vi "RasterScanXY.vi"(4 "Scanning parameters":T1) -> (1 "X,Y AO Waveforms":waveform(dbl)[](array[waveform]))   [LabVIEW 2015]
doc: "DESCRIPTION:\nThis example generates a sinewave analog output waveform on the board specified. It is an example of the simplest form of continuous waveform generation. \nA sine wave is computed using the sine trig function in a for loop. The analog output channel and buffer is initialized (AO Config), the waveform written to the the waveform buffer (AO Write) and waveform generation is initiated at the specified update rate (AO Start).\n\n\nINSTRUCTIONS:\n1. Specify device, channels, and update rate.\n2. If you want the waveform to be regenerated indefinitely, set cycles to generate to 0. Otherwise, specify the cycles to generate as a positive number. \n3. Run the VI. You will see the number of cycles generated in the cycles done indicator.\n4. If no error occurred, the example waits in a while loop for the stop button to be pressed or the requested number of buffer iterations to be completed. When either condition occurs, AO Clear stops the wavefrom generation.\n\n\nKEY PARAMETERS:\n* AO Config: device, channel\n* AO Write: (sinewave data)\n* AO Start: update rate, cycles to generate\n\n \nI/O CONNECTIONS OVERVIEW:\nConnect the I/O connector pin of the specified analog output channel to an external device (e.g. oscilloscope).\n\n\nModification Ideas:\n- For multiple channel waveform generation:\nSimply compute waveforms for other channels and collect them in a 2D array - one row for each channel. Then transpose the 2D array before connecting to AO Write. Enter the multiple channels in the \"channel\" control.\n\n- To change the waveform during generation:\nAO Write can also be used in the loop to update the waveform buffer. See the Function Generator example."
panel:
  # "this correspondes to channel \n\"0\" in stage"
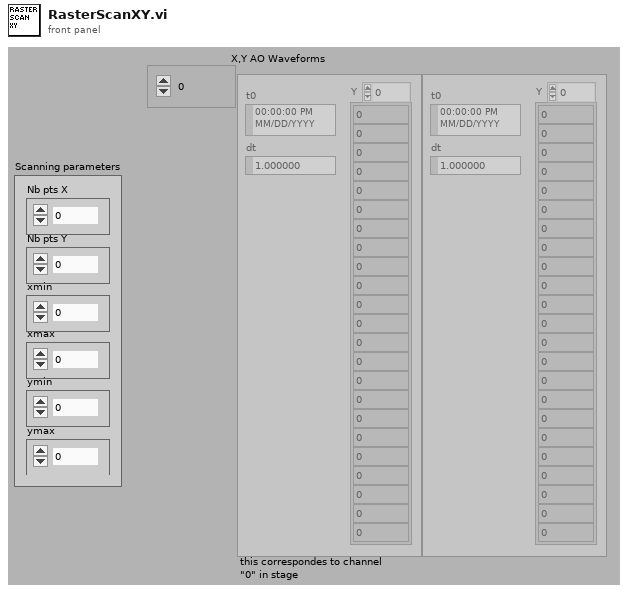
[diagram p1: front panel]
types:
  T1 = cluster{"Nb pts X":u32, "Nb pts Y":u32, "xmin":dbl, "xmax":dbl, "ymin":dbl, "ymax":dbl}
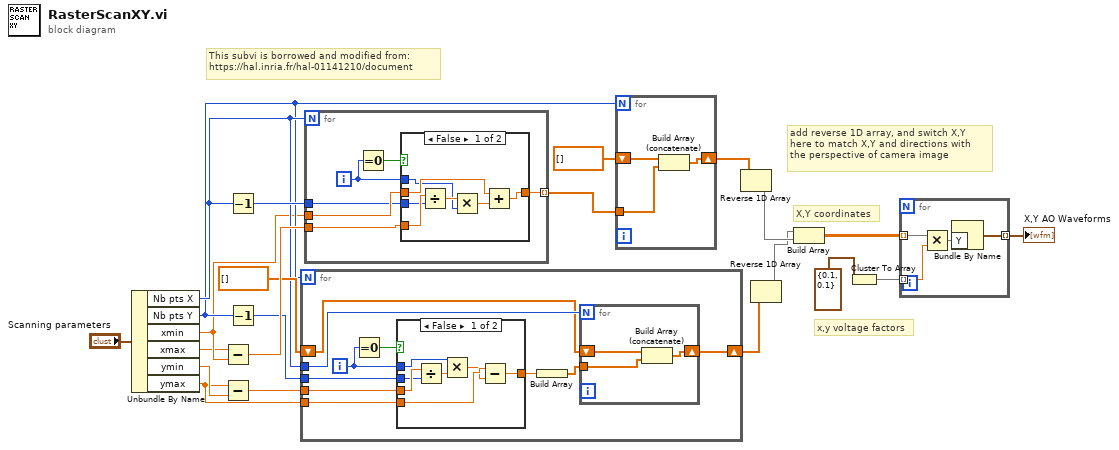
[diagram p0: block diagram]
diagram:
  # "This subvi is borrowed and modified from:  \nhttps://hal.inria.fr/hal-01141210/document"
  # "add reverse 1D array, and switch X,Y \nhere to match X,Y and directions with \nthe perspective of camera image"
  # "x,y voltage factors"
  # "X,Y coordinates"
  n1 = Unbundle By Name("Scanning parameters") -> ("Nb pts X"=w15:u32, "Nb pts Y"=w14:u32, "xmin"=w13:dbl, "xmax"=w12:dbl, "ymin"=w11:dbl, "ymax"=w10:dbl)
  n2 = Subtract(x=w12, y=w13) -> (x-y=w22:dbl)
  n3 = Subtract(x=w10, y=w11) -> (x-y=w18:dbl)
  n4 = Decrement(x=w15) -> (x-1=w21:u32)
  n5 = Decrement(x=w14) -> (x-1=w17:u32)
  n6 = for {
    N: w14 -> [_]
    tunnel: w10 -> [w31]
    tunnel: w18 -> [w30]
    tunnel: w17 -> [w29]
    tunnel: w15 -> [w26]
    shift-right: [w24] -> w4
    shift-left: dbl[] [] -> [w23]
    i -> [w28]
    n7 = Equal To 0?(x=w28) -> (x = 0?=w32:bool)
    n8 = case shown="False" w32 {
      tunnel: w31 -> [w42 w43]
      tunnel: [w38 w43] -> w27
      tunnel: w30 -> [w41 _]
      tunnel: w29 -> [w40 _]
      tunnel: w28 -> [w36 _]
      frame False {
        n9 = Divide(x=w41, y=w40) -> (x/y=w37:dbl)
        n10 = Multiply(x=w36, y=w37) -> (x*y=w39:dbl)
        n11 = Subtract(x=w42, y=w39) -> (x-y=w38:dbl)
      }
      frame True {
      }
    }
    n12 = Build Array(w27) -> (w25:dbl[])
    n13 = for {
      N: w26 -> [_]
      shift-right: [w33] -> w24
      shift-left: w23 -> [w35]
      tunnel: w25 -> [w34]
      n14 = Build Array (concatenate)(w35, w34) -> (w33:dbl[])
    }
  }
  n15 = for {
    N: w15 -> [_]
    tunnel: w13 -> [w47]
    tunnel: [w48] -> w20 mode=indexing
    tunnel: w22 -> [w46]
    tunnel: w21 -> [w45]
    i -> [w44]
    n16 = Equal To 0?(x=w44) -> (x = 0?=w49:bool)
    n17 = case shown="False" w49 {
      tunnel: w47 -> [w56 w57]
      tunnel: [w50 w57] -> w48
      tunnel: w46 -> [w55 _]
      tunnel: w45 -> [w54 _]
      tunnel: w44 -> [w52 _]
      frame False {
        n18 = Divide(x=w55, y=w54) -> (x/y=w53:dbl)
        n19 = Multiply(x=w53, y=w52) -> (x*y=w51:dbl)
        n20 = Add(x=w56, y=w51) -> (x+y=w50:dbl)
      }
      frame True {
      }
    }
  }
  n21 = for {
    N: w14 -> [_]
    shift-right: [w59] -> w3
    shift-left: dbl[] [] -> [w60]
    tunnel: w20 -> [w58]
    n22 = Build Array (concatenate)(w60, w58) -> (w59:dbl[])
  }
  n23 = Reverse 1D Array(array=w3) -> (reversed array=w2:dbl[])
  n24 = Reverse 1D Array(array=w4) -> (reversed array=w1:dbl[])
  n25 = Build Array(w1, w2) -> (w6:dbl[][])
  n26 = Cluster To Array(cluster=cluster{"XFactor":dbl, "YFactor":dbl} {"XFactor"=0.1, "YFactor"=0.1} ("VoltageFactors")) -> (array=w8:dbl[])
  n27 = for {
    tunnel: w8 -> [w63] mode=indexing
    tunnel: w6 -> [w64] mode=indexing
    tunnel: [w61] -> w9 mode=indexing
    n28 = Multiply(x=w64, y=w63) -> (x*y=w62:dbl[])
    n29 = Bundle By Name("Y"=w62) -> (w61:waveform(dbl))  [unwired: 1 in]
  }
  "X,Y AO Waveforms" <- w9
